vi "niusrprios Configure Signal (Common).vi"(0 "niUsrpRio Session":T3={"FPGA Interface"=refnum, "RIO Interface Number"=0, "Data Clock Rate"=0, "FPGA Data Clock Rate"=0, "Global Settings Register Bus"=refnum, "Radio 0 Settings Register Bus"=refnum, "Radio 1 Settings Register Bus"=refnum, "Radio Settings Bus Semaphore"=refnum, "DB Queues"=[], "Characterization Data Valid?"=FALSE, "EEPROM Header"={"Checksum"=0, "Product Code"=0, "Hardware Current Version"=0, "Hardware Oldest Compatible Version"=0, "EEPROM Map Current Version"=0, "EEPROM Map Oldest Compatible Version"=0, "User Password"="", "Pointer to Factory Header"=0, "Pointer to User Header"=0, "Recommended Interval"=0, "Number of Reserved Bytes"=9, "Number of Daughterboards"=0, "Daughterboard IDs"=[], "Daughterboard Serial Numbers"=[]}, "Device Data Header"={"Checksum"=0, "Number of Channels"=0, "Number of Gain Settings"=[], "Pointer to Characterization Data"=[], "Number of Reserved Bytes"=27, "Number of Frequencies"=[]}, "EEPROM Characterization Header"={"Checksum"=0, "Date"=timestamp(0 s since 1904-01-01), "Temperature"=0.0, "Misc. Info"="", "Pointer to Device Data Header"=0, "Number of Reserved Bytes"=28}, "Characterization Data"=[], "FPGA Current Version"=0, "FPGA Oldest Compatible Version"=0, "Fixed Logic Current Version"=0, "Fixed Logic Oldest Compatible Version"=0, "FPGA Radio Settings Bus Current Version"=0, "FPGA Radio Settings Bus Oldest Compatible Version"=0, "FPGA Board Config Current Version"=0, "FPGA Board Config Oldest Compatible Version"=0, "Daughterboard Clock Rate"=0} {"Daughterboard Clock Rate" format="%#.3pHz"; "FPGA Data Clock Rate" format="%#.3pHz"; "Data Clock Rate" format="%#.3pHz"; "Characterization Data"."Frequencies [Hz]" format="%#_6p"; "EEPROM Characterization Header"."Pointer to Device Data Header" format="%x"; "EEPROM Characterization Header"."Checksum" format="%x"; "Device Data Header"."Pointer to Characterization Data" format="%x"; "Device Data Header"."Checksum" format="%x"; "EEPROM Header"."Pointer to User Header" format="%x"; "EEPROM Header"."Pointer to Factory Header" format="%x"; "EEPROM Header"."Product Code" format="%x"; "EEPROM Header"."Checksum" format="%x"}, 1 "scope":string(combo)="rx", 2 "Correct Impairments?":bool=TRUE, 5 "signal parameters":T2={"gain/level"=0.0, "sample rate [S/s]"=10000000.0, "frequency [Hz]"=2450000000.0, "LO frequency [Hz]"=-1.0, "active antenna"="RX1"} {"LO frequency [Hz]" format="%#.3pHz"; "frequency [Hz]" format="%#.3pHz"; "sample rate [S/s]" min=1.0 max=250000000.0 format="%#.3pS/s"}, 7 "Configure Signal Mode":T1, 11 "error in":errorcluster) -> (4 "niUsrpRio Session (out)":T3={"FPGA Interface"=refnum, "RIO Interface Number"=0, "Data Clock Rate"=0, "FPGA Data Clock Rate"=0, "Global Settings Register Bus"=refnum, "Radio 0 Settings Register Bus"=refnum, "Radio 1 Settings Register Bus"=refnum, "Radio Settings Bus Semaphore"=refnum, "DB Queues"=[], "Characterization Data Valid?"=FALSE, "EEPROM Header"={"Checksum"=0, "Product Code"=0, "Hardware Current Version"=0, "Hardware Oldest Compatible Version"=0, "EEPROM Map Current Version"=0, "EEPROM Map Oldest Compatible Version"=0, "User Password"="", "Pointer to Factory Header"=0, "Pointer to User Header"=0, "Recommended Interval"=0, "Number of Reserved Bytes"=9, "Number of Daughterboards"=0, "Daughterboard IDs"=[], "Daughterboard Serial Numbers"=[]}, "Device Data Header"={"Checksum"=0, "Number of Channels"=0, "Number of Gain Settings"=[], "Pointer to Characterization Data"=[], "Number of Reserved Bytes"=27, "Number of Frequencies"=[]}, "EEPROM Characterization Header"={"Checksum"=0, "Date"=timestamp(0 s since 1904-01-01), "Temperature"=0.0, "Misc. Info"="", "Pointer to Device Data Header"=0, "Number of Reserved Bytes"=28}, "Characterization Data"=[], "FPGA Current Version"=0, "FPGA Oldest Compatible Version"=0, "Fixed Logic Current Version"=0, "Fixed Logic Oldest Compatible Version"=0, "FPGA Radio Settings Bus Current Version"=0, "FPGA Radio Settings Bus Oldest Compatible Version"=0, "FPGA Board Config Current Version"=0, "FPGA Board Config Oldest Compatible Version"=0, "Daughterboard Clock Rate"=0} {"Daughterboard Clock Rate" format="%#.3pHz"; "FPGA Data Clock Rate" format="%#.3pHz"; "Data Clock Rate" format="%#.3pHz"; "Characterization Data"."Frequencies [Hz]" format="%#_6p"; "EEPROM Characterization Header"."Pointer to Device Data Header" format="%x"; "EEPROM Characterization Header"."Checksum" format="%x"; "Device Data Header"."Pointer to Characterization Data" format="%x"; "Device Data Header"."Checksum" format="%x"; "EEPROM Header"."Pointer to User Header" format="%x"; "EEPROM Header"."Pointer to Factory Header" format="%x"; "EEPROM Header"."Product Code" format="%x"; "EEPROM Header"."Checksum" format="%x"}, 6 "coerced signal parameters":T2={"gain/level"=0.0, "sample rate [S/s]"=10000000.0, "frequency [Hz]"=2450000000.0, "LO frequency [Hz]"=-1.0, "active antenna"="RX1"} {"LO frequency [Hz]" format="%#.3pHz"; "frequency [Hz]" format="%#.3pHz"; "sample rate [S/s]" min=1.0 max=250000000.0 format="%#.3pS/s"}, 15 "error out":errorcluster)   [LabVIEW 2015]
doc: "Configures the DSP and signal path for the channel based on the input <B>signal parameters</B>.\n\n<B>Input Parameters</B>\n\n<B>Sample Rate</B> the requested rate, in samples per second, the signal will be sampled at.\n\n<B>Frequency</B> is the requested frequency, in hertz, to acquire the signal from/generate the signal at.\n\n<B>Level</B> is the requested power level, in dBm, of the signal.\n\n<B>Gain</B> is the requested amount of gain, in dB.\n\n<B>LO Frequency</B> is the requested frequency, in hertz, to tune the local oscillator to. The default value of -1 sets the LO to the value of the 'Frequency' input. If the value is not -1, the LO will be set to that value, and the DSP will handle the difference between the 'Frequency' and the 'LO Frequency'.\n\n<B>Active Antenna</B> is the antenna to use for this channel.\n\n<B>Correct Impairments</B> applies the correction information of the device to the signal."
uses:
  <instrlib>/niUsrpRio/Config/v1/Host/Public/niUsrpRio Session.ctl
  <instrlib>/_niInstr/Register Bus/v0/Host/Public/Register Bus Session.ctl
  <instrlib>/_niInstr/Register Bus/v0/Host/Private/Session Data.ctl
  <instrlib>/niUsrpRio/Config/v1/Host/Private/DB Queue Reference.ctl
  <instrlib>/niUsrpRio/Config/v1/Host/Private/Daughterboard Data.ctl
  <instrlib>/niUsrpRio/Config/v1/Host/Private/ATR state data.ctl
  <instrlib>/niUsrpRio/Config/v1/Host/Private/Antenna Configuration.ctl
  <instrlib>/niUsrpRio/Config/v1/Host/Private/CPLD Power Mode.ctl
  <instrlib>/niUsrpRio/Config/v1/Host/Public/EEPROM Header.ctl
  <instrlib>/niUsrpRio/Config/v1/Host/Public/EEPROM Device Data Header.ctl
  <instrlib>/niUsrpRio/Config/v1/Host/Public/EEPROM Characterization Header.ctl
  <instrlib>/niUsrpRio/Config/v1/Host/Public/Characterization Data.ctl
  <instrlib>/niUsrpRio/Config/v1/Host/Public/IQ Imbalance.ctl
  niusrprios Configure Signal Parameters.ctl
  niusrprios Configure Signal Mode.ctl
  niusrprios Streaming Xvcr FPGA Ref.ctl
  <instrlib>/_niInstr/DSP/v1/Shared/Public/IQ Impairments.ctl
  <instrlib>/_niInstr/DSP/v1/Shared/Public/IQ Gain.ctl
  <vilib>/rvi/errors/niLvFpgaAdjustHostInterfaceError.vi
  <vilib>/Utility/error.llb/Error Cluster From Error Code.vi
  <vilib>/rvi/interface/nirviReadWriteControl/nirviReadWriteControl.xnode
  <vilib>/ErrorRing/Error Ring.xnode
  NiFpgaLv.dll
  <vilib>/rvi/interface/Simulation/niFpgaSimulationCallBeginRW.vi
  <instrlib>/_niInstr/DSP/v1/Shared/niInstr DSP v1 Shared.lvlib
  <instrlib>/niUsrpRio/Config/v1/Host/niUsrpRio Config v1 Host.lvlib
  <instrlib>/_niInstr/Register Bus/v0/Host/niInstr Register Bus v0 Host.lvlib
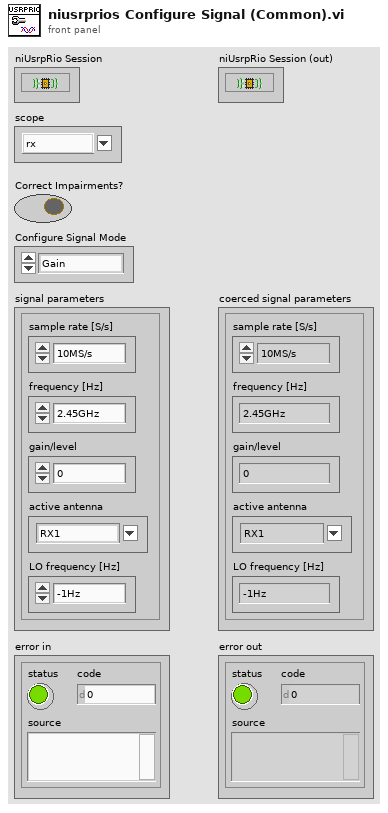
[diagram p1: front panel]
types:
  T1 = typedef "niusrprios Configure Signal Mode.ctl" = enum16{"Gain", "Level"}
  T2 = typedef "niusrprios Configure Signal Parameters.ctl" = cluster{"gain/level":dbl, "sample rate [S/s]":dbl, "frequency [Hz]":dbl, "LO frequency [Hz]":dbl, "active antenna":string}
  T3 = typedef "niUsrpRio Config v1 Host.lvlib/niUsrpRio Session.ctl" = cluster{"FPGA Interface":refnum<k20>, "RIO Interface Number":u32, "Data Clock Rate":u32, "FPGA Data Clock Rate":u32, "Global Settings Register Bus":T4, "Radio 0 Settings Register Bus":T4, "Radio 1 Settings Register Bus":T4, "Radio Settings Bus Semaphore":T5, "DB Queues":T6[], "Characterization Data Valid?":bool, "EEPROM Header":T7, "Device Data Header":T8, "EEPROM Characterization Header":T9, "Characterization Data":T10[], "FPGA Current Version":u32, "FPGA Oldest Compatible Version":u32, "Fixed Logic Current Version":u32, "Fixed Logic Oldest Compatible Version":u32, "FPGA Radio Settings Bus Current Version":u32, "FPGA Radio Settings Bus Oldest Compatible Version":u32, "FPGA Board Config Current Version":u32, "FPGA Board Config Oldest Compatible Version":u32, "Daughterboard Clock Rate":u32}
  T4 = typedef "niInstr Register Bus v0 Host.lvlib/Register Bus Session.ctl" = refnum<queue>
  T5 = typedef "Semaphore RefNum" = refnum<k1>
  T6 = typedef "niUsrpRio Config v1 Host.lvlib/DB Queue Reference.ctl" = refnum<queue>
  T7 = typedef "niUsrpRio Config v1 Host.lvlib/EEPROM Header.ctl" = cluster{"Checksum":u32, "Product Code":u16, "Hardware Current Version":u16, "Hardware Oldest Compatible Version":u16, "EEPROM Map Current Version":u16, "EEPROM Map Oldest Compatible Version":u16, "User Password":string, "Pointer to Factory Header":u32, "Pointer to User Header":u32, "Recommended Interval":u16, "Number of Reserved Bytes":i32, "Number of Daughterboards":u8, "Daughterboard IDs":u16[], "Daughterboard Serial Numbers":string[]}
  T8 = typedef "niUsrpRio Config v1 Host.lvlib/EEPROM Device Data Header.ctl" = cluster{"Checksum":u32, "Number of Channels":u8, "Number of Gain Settings":u16[], "Pointer to Characterization Data":u32[], "Number of Reserved Bytes":i32, "Number of Frequencies":u16[]}
  T9 = typedef "niUsrpRio Config v1 Host.lvlib/EEPROM Characterization Header.ctl" = cluster{"Checksum":u32, "Date":timestamp, "Temperature":sgl, "Misc. Info":string, "Pointer to Device Data Header":u32, "Number of Reserved Bytes":i32}
  T10 = typedef "niUsrpRio Config v1 Host.lvlib/Characterization Data.ctl" = cluster{"Gains[dB]":dbl[], "Frequencies [Hz]":dbl[], "IQ Imbalance Table":T11[], "Measured Gains[dB]":dbl[][]}
  T11 = typedef "niUsrpRio Config v1 Host.lvlib/IQ Imbalance.ctl" = cluster{"Gain Imbalance [linear]":dbl, "Phase Imbalance [radians]":dbl, "Offset":cdb}
  T12 = typedef "niusrprios Streaming Xvcr FPGA Ref.ctl" = refnum<k20>
  T13 = typedef "niInstr DSP v1 Shared.lvlib/IQ Impairments.ctl" = cluster{"inline gain I":fxp<+/-,18,1>, "inline gain Q":fxp<+/-,18,1>, "cross gain I":fxp<+/-,18,1>, "cross gain Q":fxp<+/-,18,1>, "pre-gain offset I":fxp<+/-,18,1>, "pre-gain offset Q":fxp<+/-,18,1>, "post-gain offset I":fxp<+/-,18,1>, "post-gain offset Q":fxp<+/-,18,1>}
  T14 = typedef "niUsrpRio Config v1 Host.lvlib/Device Subfunction.ctl" = enum16{"rx", "tx", "all"}
  T15 = typedef "niUsrpRio Config v1 Host.lvlib/RF Channel.ctl" = enum16{"0", "1", "All"}
  T16 = typedef "niInstr DSP v1 Shared.lvlib/IQ Gain.ctl" = cluster{"gain I":fxp<+/-,24,3>, "gain Q":fxp<+/-,24,3>}
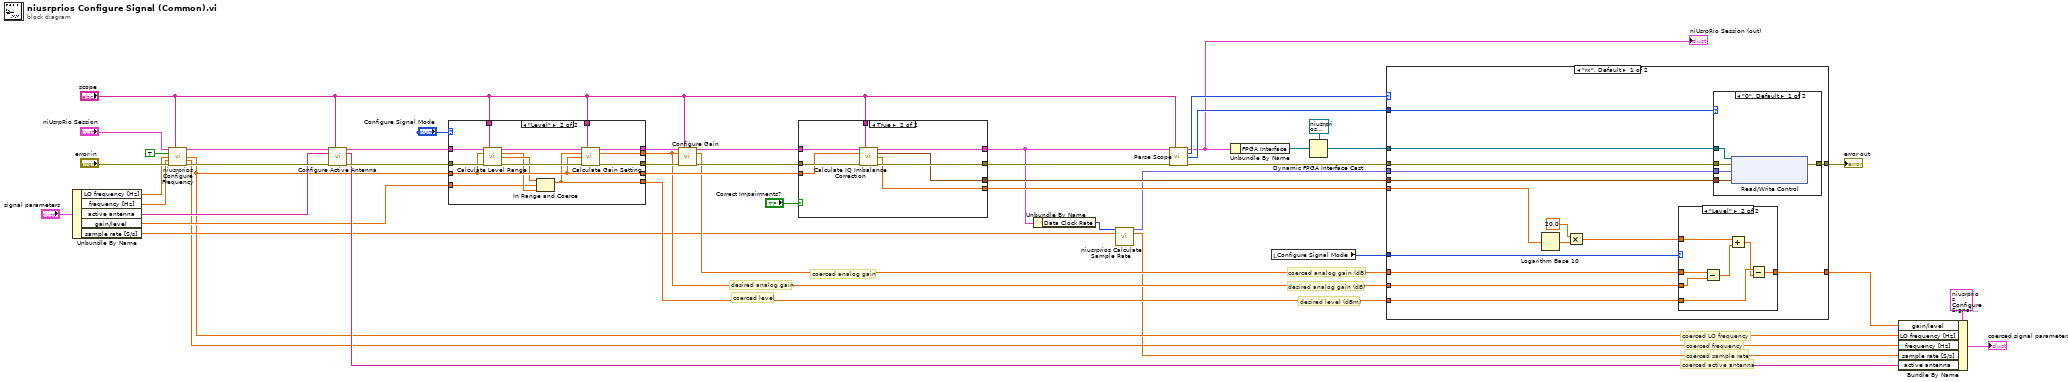
[diagram p0: block diagram]
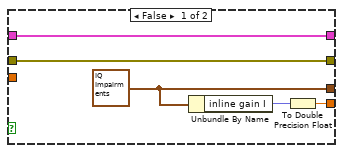
[diagram p3: hidden frame]
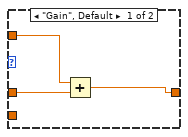
[diagram p4: hidden frame]
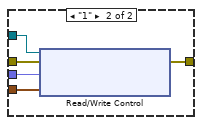
[diagram p5: hidden frame]
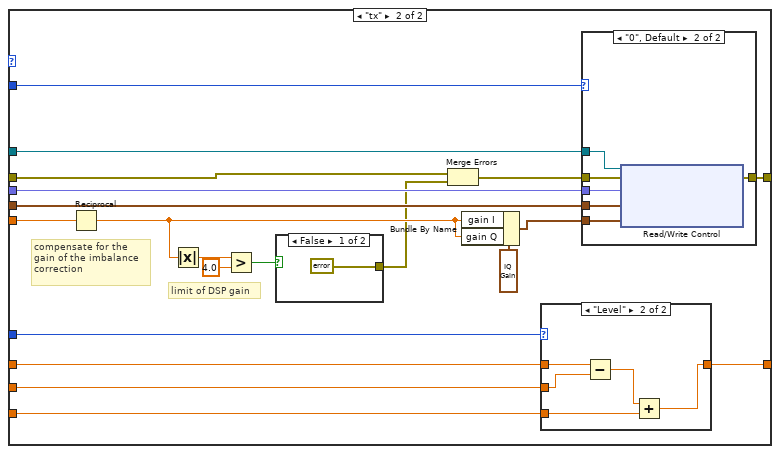
[diagram p6: hidden frame]
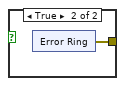
[diagram p7: hidden frame]
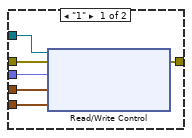
[diagram p9: hidden frame]
diagram:
  # "coerced level"
  # "desired level (dBm)"
  # "desired analog gain"
  # "desired analog gain (dB)"
  # "coerced analog gain (dB)"
  # "coerced analog gain"
  # "coerced active antenna"
  # "coerced sample rate"
  # "coerced frequency"
  # "coerced LO frequency"
  n1 = Unbundle By Name("signal parameters") -> ("LO frequency [Hz]"=w33:dbl, "frequency [Hz]"=w22:dbl, "active antenna"=w32:string, "gain/level"=w16:dbl, "sample rate [S/s]"=w2:dbl)
  n2 = call "niusrprios Configure Frequency.vi"("niUsrpRio Session"="niUsrpRio Session", "scope"="scope", "wait for lo to lock"=TRUE, "lo frequency"=w33, "frequency"=w22, "error in"="error in") -> ("niUsrpRio Session (out)"=w39:T3, "coerced lo frequency"=w14:dbl, "coerced frequency"=w1:dbl, "error out"=w38:errorcluster)  [unwired: 6 in]
  n3 = call <instrlib>:"Configure Active Antenna.vi"("niUsrpRio Session"=w39, "scope"="scope", "active antenna"=w32, "error in"=w38) -> ("niUsrpRio Session (out)"=w30:T3, "coerced active antenna"=w21:string, "error out"=w29:errorcluster)  [unwired: 9 in]
  n4 = case shown="\"Level\"" "Configure Signal Mode" {
    tunnel: w30 -> [w49 w54]
    tunnel: w29 -> [w48 w63]
    tunnel: w16 -> [w47 w55]
    tunnel: "scope" -> [_ w60]
    tunnel: [w49 w59] -> w26
    tunnel: w14 -> [w50 w61]
    tunnel: [w50 w61] -> w28
    tunnel: [w48 w64] -> w27
    tunnel: [w47 w58] -> w17
    tunnel: "scope" -> [_ w52]
    tunnel: [w47 w51] -> w11
    frame "Gain", Default {
    }
    frame "Level" {
      n5 = call <instrlib>:"Calculate Level Range.vi"("niUsrpRio Session"=w54, "scope"=w52, "frequency"=w61, "error in"=w63) -> ("niUsrpRio Session (out)"=w53:T3, "Min Level"=w56:dbl, "Max Level"=w57:dbl, "error out"=w62:errorcluster)  [unwired: 8 in]
      n6 = In Range and Coerce(upper limit=w57, x=w55, lower limit=w56) -> (coerced(x)=w51:dbl)  [unwired: 1 out]
      n7 = call <instrlib>:"Calculate Gain Setting.vi"("niUsrpRio Session"=w53, "scope"=w60, "level"=w51, "frequency"=w61, "error in"=w62) -> ("niUsrpRio Session (out)"=w59:T3, "gain"=w58:dbl, "error out"=w64:errorcluster)  [unwired: 8 in]
    }
  }
  n8 = call <instrlib>:"Configure Gain.vi"("niUsrpRio Session"=w26, "scope"="scope", "gain"=w17, "Error In"=w27) -> ("niUsrpRio Session (out)"=w25:T3, "coerced gain"=w18:dbl, "Error Out"=w24:errorcluster)  [unwired: 9 in]
  n9 = case shown="True" "Correct Impairments?" {
    tunnel: w24 -> [w68 w76]
    tunnel: w25 -> [w69 w77]
    tunnel: "scope" -> [_ w75]
    tunnel: [w69 w74] -> w6
    tunnel: [w68 w73] -> w7
    tunnel: [w65 w72] -> w36
    tunnel: [w66 w70] -> w35
    tunnel: w28 -> [_ w71]
    frame False {
      w65 = T13 {"inline gain I"=0.9999923706054688, "inline gain Q"=0.9999923706054688, "cross gain I"=0.0, "cross gain Q"=0.0, "pre-gain offset I"=0.0, "pre-gain offset Q"=0.0, "post-gain offset I"=0.0, "post-gain offset Q"=0.0} ("impairment control")
      n10 = Unbundle By Name(w65) -> ("inline gain I"=w67:fxp<+/-,18,1>)
      n11 = To Double Precision Float(number=w67) -> (double precision float=w66:dbl)
    }
    frame True {
      n12 = call <instrlib>:"Calculate IQ Imbalance Correction.vi"("niUsrpRio Session"=w77, "scope"=w75, "frequency"=w71, "error in"=w76) -> ("niUsrpRio Session (out)"=w74:T3, "IQ imbalance correction"=w72:T13, "correction gain"=w70:dbl, "error out"=w73:errorcluster)  [unwired: 8 in]
    }
  }
  n13 = Unbundle By Name(w6) -> ("Data Clock Rate"=w5:u32)
  n14 = call "niusrprios Calculate Sample Rate.vi"("data clock rate"=w5, "sample rate"=w2) -> ("decimation sample rate"=w3:fxp<+,48,1>, "coerced sample rate"=w4:dbl)  [unwired: 12 in]
  n15 = call <instrlib>:"Parse Scope.vi"("niUsrpRio Session"=w6, "scope"="scope", "error in"=w7) -> ("niUsrpRio Session (out)"=w41:T3, "Device Subfunction"=w43:T14, "Device Subfunction Channel"=w42:T15, "error out"=w40:errorcluster)  [unwired: 4 in, 5 out]
  "niUsrpRio Session (out)" <- w41
  n16 = Unbundle By Name(w41) -> ("FPGA Interface"=w10:refnum<k20>)
  n17 = local read "Configure Signal Mode"() -> (w19:T1)
  n18 = Dynamic FPGA Interface Cast(Session In=T12 refnum ("FPGA VI Reference Out"), Type=w10) -> (Session Out=w9:T12)
  n19 = case shown="\"rx\", Default" w43 {
    tunnel: w3 -> [w92 w132]
    tunnel: w9 -> [w91 w113]
    tunnel: [w90 w131] -> w46
    tunnel: w40 -> [w89 w130]
    tunnel: w36 -> [w88 w129]
    tunnel: w42 -> [w87 w128]
    tunnel: w35 -> [w81 w126]
    tunnel: w19 -> [w85 w124]
    tunnel: w18 -> [w86 w123]
    tunnel: [w84 w122] -> w15
    tunnel: w17 -> [w82 w121]
    tunnel: w11 -> [w83 w120]
    frame "rx", Default {
      n20 = Logarithm Base 10(1:w81) -> (0:w79:dbl)
      n21 = Multiply(x=20.0, y=w79) -> (x*y=w78:dbl)
      n22 = case shown="\"Level\"" w85 {
        tunnel: w86 -> [w94 w102]
        tunnel: [w93 w96] -> w84
        tunnel: w82 -> [_ w101]
        tunnel: w83 -> [_ w98]
        tunnel: w78 -> [w95 w100]
        frame "Gain", Default {
          n23 = Add(x=w95, y=w94) -> (x+y=w93:dbl)
        }
        frame "Level" {
          n24 = Subtract(x=w102, y=w101) -> (x-y=w99:dbl)
          n25 = Add(x=w100, y=w99) -> (x+y=w97:dbl)
          n26 = Subtract(x=w98, y=w97) -> (x-y=w96:dbl)
        }
      }
      n27 = case shown="\"0\", Default" w87 {
        tunnel: w92 -> [w105 w112]
        tunnel: [w103 w111] -> w90
        tunnel: w89 -> [w107 w110]
        tunnel: w91 -> [w106 w109]
        tunnel: w88 -> [w104 w108]
        frame "0", Default {
          n28 = xnode "Read/Write Control"("FPGA VI Reference In"=w106, "error in"=w107, "rx.output sample rate"=w105, "rx 0.impairments"=w104) -> ("error out"=w103:errorcluster)  [unwired: 1 out]
        }
        frame "1" {
          n29 = xnode "Read/Write Control"("FPGA VI Reference In"=w109, "error in"=w110, "rx.output sample rate"=w112, "rx 1.impairments"=w108) -> ("error out"=w111:errorcluster)  [unwired: 1 out]
        }
      }
    }
    frame "tx" {
      # "limit of DSP gain"
      # "compensate for the\ngain of the imbalance\ncorrection"
      n30 = Reciprocal(x=w126) -> (1/x=w118:dbl)
      n31 = Absolute Value(x=w118) -> (abs(x)=w116:dbl)
      n32 = Greater?(x=w116, y=4.0) -> (0:w119:bool)
      n33 = case shown="False" w119 {
        tunnel: [errorcluster {"status"=FALSE, "code"=0, "source"=""} ("error constant") w134] -> w114
        frame False {
        }
        frame True {
          n34 = xnode "Error Ring"() -> ("error out"=w134:errorcluster)
        }
      }
      n35 = Merge Errors(w130, w114) -> (w115:errorcluster)
      n36 = Bundle By Name(cluster=T16 {"gain I"=1.0, "gain Q"=1.0} ("gain"), "gain I"=w118, "gain Q"=w118) -> (w125:T16)
      n37 = case shown="\"Level\"" w124 {
        tunnel: w123 -> [w140 w145]
        tunnel: [w140 w141] -> w122
        tunnel: w121 -> [_ w144]
        tunnel: w120 -> [_ w143]
        frame "Gain", Default {
        }
        frame "Level" {
          n38 = Subtract(x=w145, y=w144) -> (x-y=w142:dbl)
          n39 = Add(x=w142, y=w143) -> (x+y=w141:dbl)
        }
      }
      n40 = case shown="\"0\", Default" w128 {
        tunnel: w132 -> [w151 w157]
        tunnel: [w150 w156] -> w131
        tunnel: w115 -> [w149 w155]
        tunnel: w113 -> [w148 w154]
        tunnel: w129 -> [w147 w153]
        tunnel: w125 -> [w146 w152]
        frame "1" {
          n41 = xnode "Read/Write Control"("FPGA VI Reference In"=w148, "error in"=w149, "tx.input sample rate"=w151, "tx 1.impairments"=w147, "tx 1.gain"=w146) -> ("error out"=w150:errorcluster)  [unwired: 1 out]
        }
        frame "0", Default {
          n42 = xnode "Read/Write Control"("FPGA VI Reference In"=w154, "error in"=w155, "tx.input sample rate"=w157, "tx 0.impairments"=w153, "tx 0.gain"=w152) -> ("error out"=w156:errorcluster)  [unwired: 1 out]
        }
      }
    }
  }
  "error out" <- w46
  n43 = Bundle By Name(cluster=T2 {"gain/level"=0.0, "sample rate [S/s]"=10000000.0, "frequency [Hz]"=2450000000.0, "LO frequency [Hz]"=-1.0, "active antenna"="RX1"} ("coerced signal parameters"), "gain/level"=w15, "LO frequency [Hz]"=w14, "frequency [Hz]"=w1, "sample rate [S/s]"=w4, "active antenna"=w21) -> (→"coerced signal parameters":T2)
